vi "GetNodesGlobal.vi"(7 "GBL VI Name":string, 10 "All Objects[] + Nodes[]":refnum<vi>[](array[refnum]), 11 "Caller VI Name":string) -> (0 "WriteGlobal?":bool, 1 "WriteGlobal":string, 2 "ReadGlobal?":bool, 3 "ReadGlobal":string)   [LabVIEW 2020]
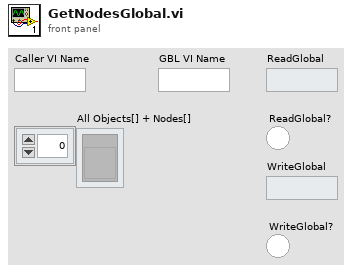
[diagram p1: front panel]
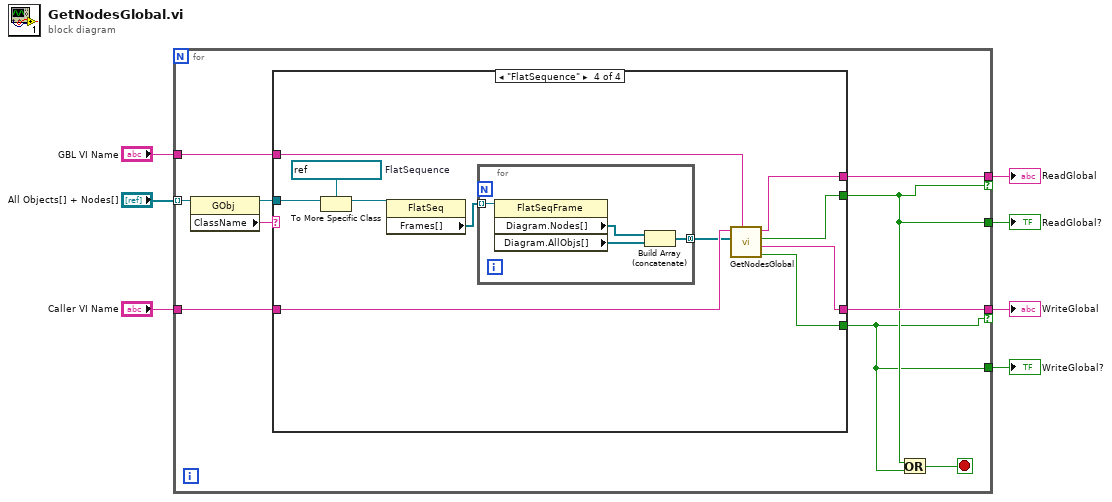
[diagram p0: block diagram]
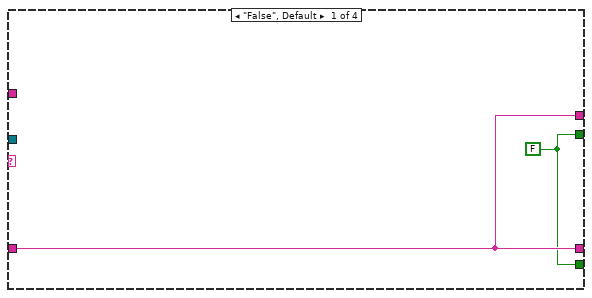
[diagram p2: hidden frame]
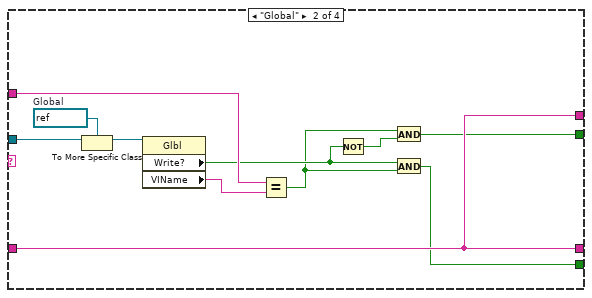
[diagram p3: hidden frame]
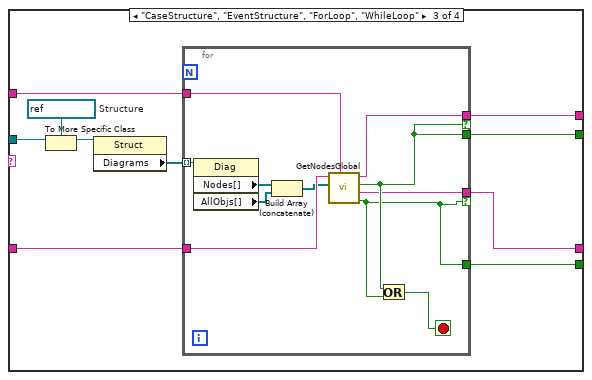
[diagram p4: hidden frame]
diagram:
  n1 = for {
    tunnel: "All Objects[] + Nodes[]" -> [w17] mode=indexing
    tunnel: [w11] -> w7 if=w8
    tunnel: [w12] -> w6 if=w9
    tunnel: "Caller VI Name" -> [w15]
    tunnel: "GBL VI Name" -> [w14]
    tunnel: [w9] -> w1
    tunnel: [w8] -> w2
    stop <- w10 stop-if-true
    n2 = property class="GObj"(reference=w17) -> (reference out=w16:refnum<vi>, "ClassName"=w13:string)  [unwired: 1 in, 1 out]
    n3 = case shown="\"FlatSequence\"" w13 {
      tunnel: w16 -> [_ w28 w40 w62]
      tunnel: w15 -> [w19 w25 w36 w59]
      tunnel: w14 -> [_ w26 w35 w58]
      tunnel: [w19 w25 w34 w57] -> w12
      tunnel: [w19 w25 w32 w55] -> w11
      tunnel: [w18 w21 w33 w56] -> w9
      tunnel: [w18 w20 w31 w54] -> w8
      frame "False", Default {
        w18 = FALSE
      }
      frame "Global" {
        w30 = refnum<vi> refnum  # Global
        n4 = To More Specific Class(target class=w30, reference=w28) -> (specific class reference=w29:refnum<vi>)  [unwired: 1 in, 1 out]
        n5 = property class="Glbl"(reference=w29) -> ("Write?"=w23:bool, "VIName"=w27:string)  [unwired: 1 in, 2 out]
        n6 = Equal?(x=w26, y=w27) -> (x = y?=w22:bool)
        n7 = Not(x=w23) -> (.not. x?=w24:bool)
        n8 = And(x=w22, y=w24) -> (x .and. y?=w21:bool)
        n9 = And(x=w23, y=w22) -> (x .and. y?=w20:bool)
      }
      frame "CaseStructure", "EventStructure", "ForLoop", "WhileLoop" {
        w39 = refnum<vi> refnum  # Structure
        n10 = To More Specific Class(target class=w39, reference=w40) -> (specific class reference=w38:refnum<vi>)  [unwired: 1 in, 1 out]
        n11 = property class="Struct"(reference=w38) -> ("Diagrams"=w37:refnum<vi>[])  [unwired: 1 in, 2 out]
        n12 = for {
          tunnel: w37 -> [w51] mode=indexing
          tunnel: w36 -> [w49]
          tunnel: w35 -> [w48]
          tunnel: [w47] -> w34 if=w45
          tunnel: [w45] -> w33
          tunnel: [w44] -> w32 if=w43
          tunnel: [w43] -> w31
          stop <- w46 stop-if-true
          n13 = property class="Diag"(reference=w51) -> ("Nodes[]"=w50:refnum<vi>[], "AllObjs[]"=w41:refnum<vi>[])  [unwired: 1 in, 2 out]
          n14 = Build Array (concatenate)(w50, w41) -> (w42:refnum<vi>[])
          n15 = call "GetNodesGlobal.vi"("GBL VI Name"=w48, "All Objects[] + Nodes[]"=w42, "Caller VI Name"=w49) -> ("WriteGlobal?"=w43:bool, "WriteGlobal"=w44:string, "ReadGlobal?"=w45:bool, "ReadGlobal"=w47:string)  [unwired: 5 in]
          n16 = Or(x=w45, y=w43) -> (x .or. y?=w46:bool)
        }
      }
      frame "FlatSequence" {
        w61 = refnum<vi> refnum  # FlatSequence
        n17 = To More Specific Class(target class=w61, reference=w62) -> (specific class reference=w60:refnum<vi>)  [unwired: 1 in, 1 out]
        n18 = property class="FlatSeq"(reference=w60) -> ("Frames[]"=w53:refnum<vi>[])  [unwired: 1 in, 2 out]
        n19 = for {
          tunnel: w53 -> [w66] mode=indexing
          tunnel: [w63] -> w52 mode=concatenating
          n20 = property class="FlatSeqFrame"(reference=w66) -> ("Diagram.Nodes[]"=w65:refnum<vi>[], "Diagram.AllObjs[]"=w64:refnum<vi>[])  [unwired: 1 in, 2 out]
          n21 = Build Array (concatenate)(w65, w64) -> (w63:refnum<vi>[])
        }
        n22 = call "GetNodesGlobal.vi"("GBL VI Name"=w58, "All Objects[] + Nodes[]"=w52, "Caller VI Name"=w59) -> ("WriteGlobal?"=w54:bool, "WriteGlobal"=w55:string, "ReadGlobal?"=w56:bool, "ReadGlobal"=w57:string)  [unwired: 5 in]
      }
    }
    n23 = Or(x=w9, y=w8) -> (x .or. y?=w10:bool)
  }
  "WriteGlobal" <- w7
  "ReadGlobal" <- w6
  "WriteGlobal?" <- w2
  "ReadGlobal?" <- w1
